vi "PH_ImageOperator.evt call set Analysis Method.vi"(0 "i ref in":refnum<vi>, 1 "Instance":string, 2 "Method":bool, 3 "Steps (3)":i32=3, 4 "Factor for ROI (3)":i32=3, 5 "error in (no error)":errorcluster) -> (14 "i ref out":refnum<vi>, 19 "error out":errorcluster)   [LabVIEW 2014, in "PH_ImageOperator.lvlib"]
doc: "This VI calls the event case \"SetAnalysisMethod\" by a simple call."
uses:
  PH_ImageOperator.lvlib
  CS_Core/CSSystem/CoreLib/CoreLib.int 2 byte array.vi
  CS_Core/CSSystem/CoreLib/CoreLib.short 2 byte array.vi
  CS_Core/CSSystem/CoreLib/CoreLib.lvlib
  CS_Core/BaseProcess/BaseProcess.lvlib
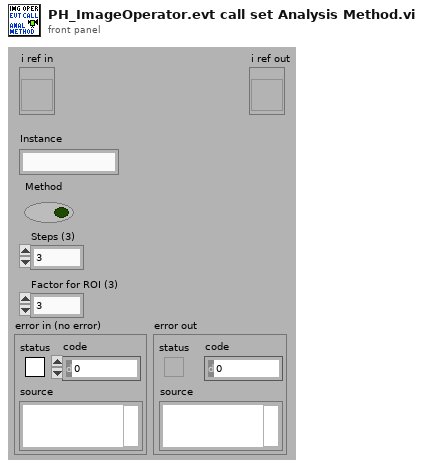
[diagram p1: front panel]
types:
  T1 = typedef "CoreDefs.rawDataType.ctl" = i8[]
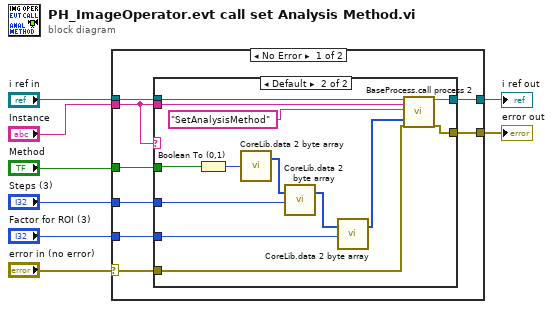
[diagram p0: block diagram]
diagram:
  n1 = case shown="No Error" "error in (no error)" {
    selector: "error in (no error)" -> [w12 w32]
    tunnel: [w16 w33] -> w8
    tunnel: [w15 w32] -> w7
    tunnel: "i ref in" -> [w14 w33]
    tunnel: "Instance" -> [w11 _]
    tunnel: "Method" -> [w13 _]
    tunnel: "Steps (3)" -> [w10 _]
    tunnel: "Factor for ROI (3)" -> [w9 _]
    frame No Error {
      n2 = case shown="Default" w11 {
        tunnel: [w18 w30] -> w16
        tunnel: [w17 w29] -> w15
        tunnel: w14 -> [w18 w28]
        tunnel: w11 -> [_ w27]
        tunnel: w13 -> [_ w19]
        tunnel: w12 -> [w17 w26]
        tunnel: w10 -> [_ w21]
        tunnel: w9 -> [_ w20]
        frame "N/A" {
        }
        frame Default {
          n3 = Boolean To (0,1)(Boolean=w19) -> (0, 1=w25:i16)
          n4 = call-poly "CoreLib.data 2 byte array.vi"("i16"=w25) -> ("byteArray out"=w23:T1)  [unwired: 18 in]
          n5 = call-poly "CoreLib.data 2 byte array.vi"("byteArray"=w23, "i32"=w21) -> ("byteArray out"=w24:T1)  [unwired: 17 in]
          n6 = call-poly "CoreLib.data 2 byte array.vi"("byteArray"=w24, "i32"=w20) -> ("byteArray out"=w22:T1)  [unwired: 17 in]
          n7 = call "BaseProcess.call process 2.vi"("i ref in"=w28, "Object"=w27, "Selector"="SetAnalysisMethod", "Data"=w22, "error in (no error)"=w26) -> ("i ref out"=w30:refnum<vi>, "error out"=w29:errorcluster)  [unwired: 13 in]
        }
      }
    }
    frame Error {
    }
  }
  "i ref out" <- w8
  "error out" <- w7
